vi "run.vi"(8 "error in (no error)":errorcluster, 11 "Protocol_Logging in":refnum<class "Protocol_Logging.lvclass">) -> (0 "error out":errorcluster, 3 "Protocol_Logging out":refnum<class "Protocol_Logging.lvclass">)   [LabVIEW 2011, in "Protocol_Logging.lvclass"]
uses:
  Protocol_Logging.lvclass
  protocol_Generic/Protocol_Generic.lvclass
panel:
  out "Waveform Graph":dbl[][](graph)
  out "path":path
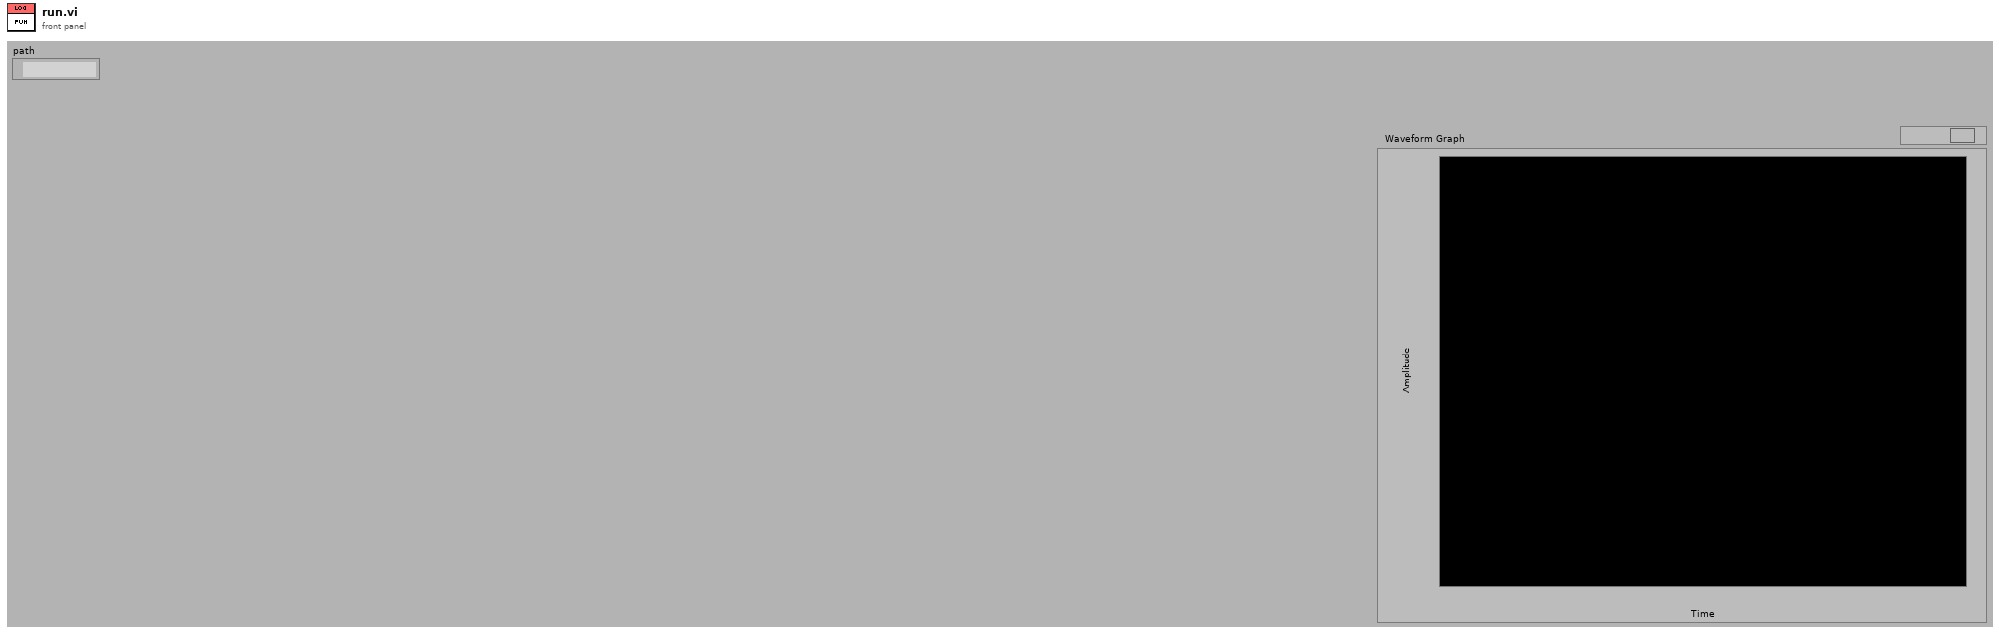
[diagram p1: front panel]
types:
  T1 = cluster{"channel0ConversionFactor":dbl, "channel1ConversionFactor":dbl, "channel2ConversionFactor":dbl}
  T2 = cluster{"Axis Information":cluster{"Device ID":i32, "Device Name":string, "Device Type":i32}[], "Axis Selector":i32[], "Control Modes out":u16[], "error out":errorcluster, "Channel Data":cluster{"Name":string, "Type":i32, "SI Full Scale":dbl, "Full Scale":dbl, "Units String":string, "Display Format":string, "Gauge Length":dbl}[][]}
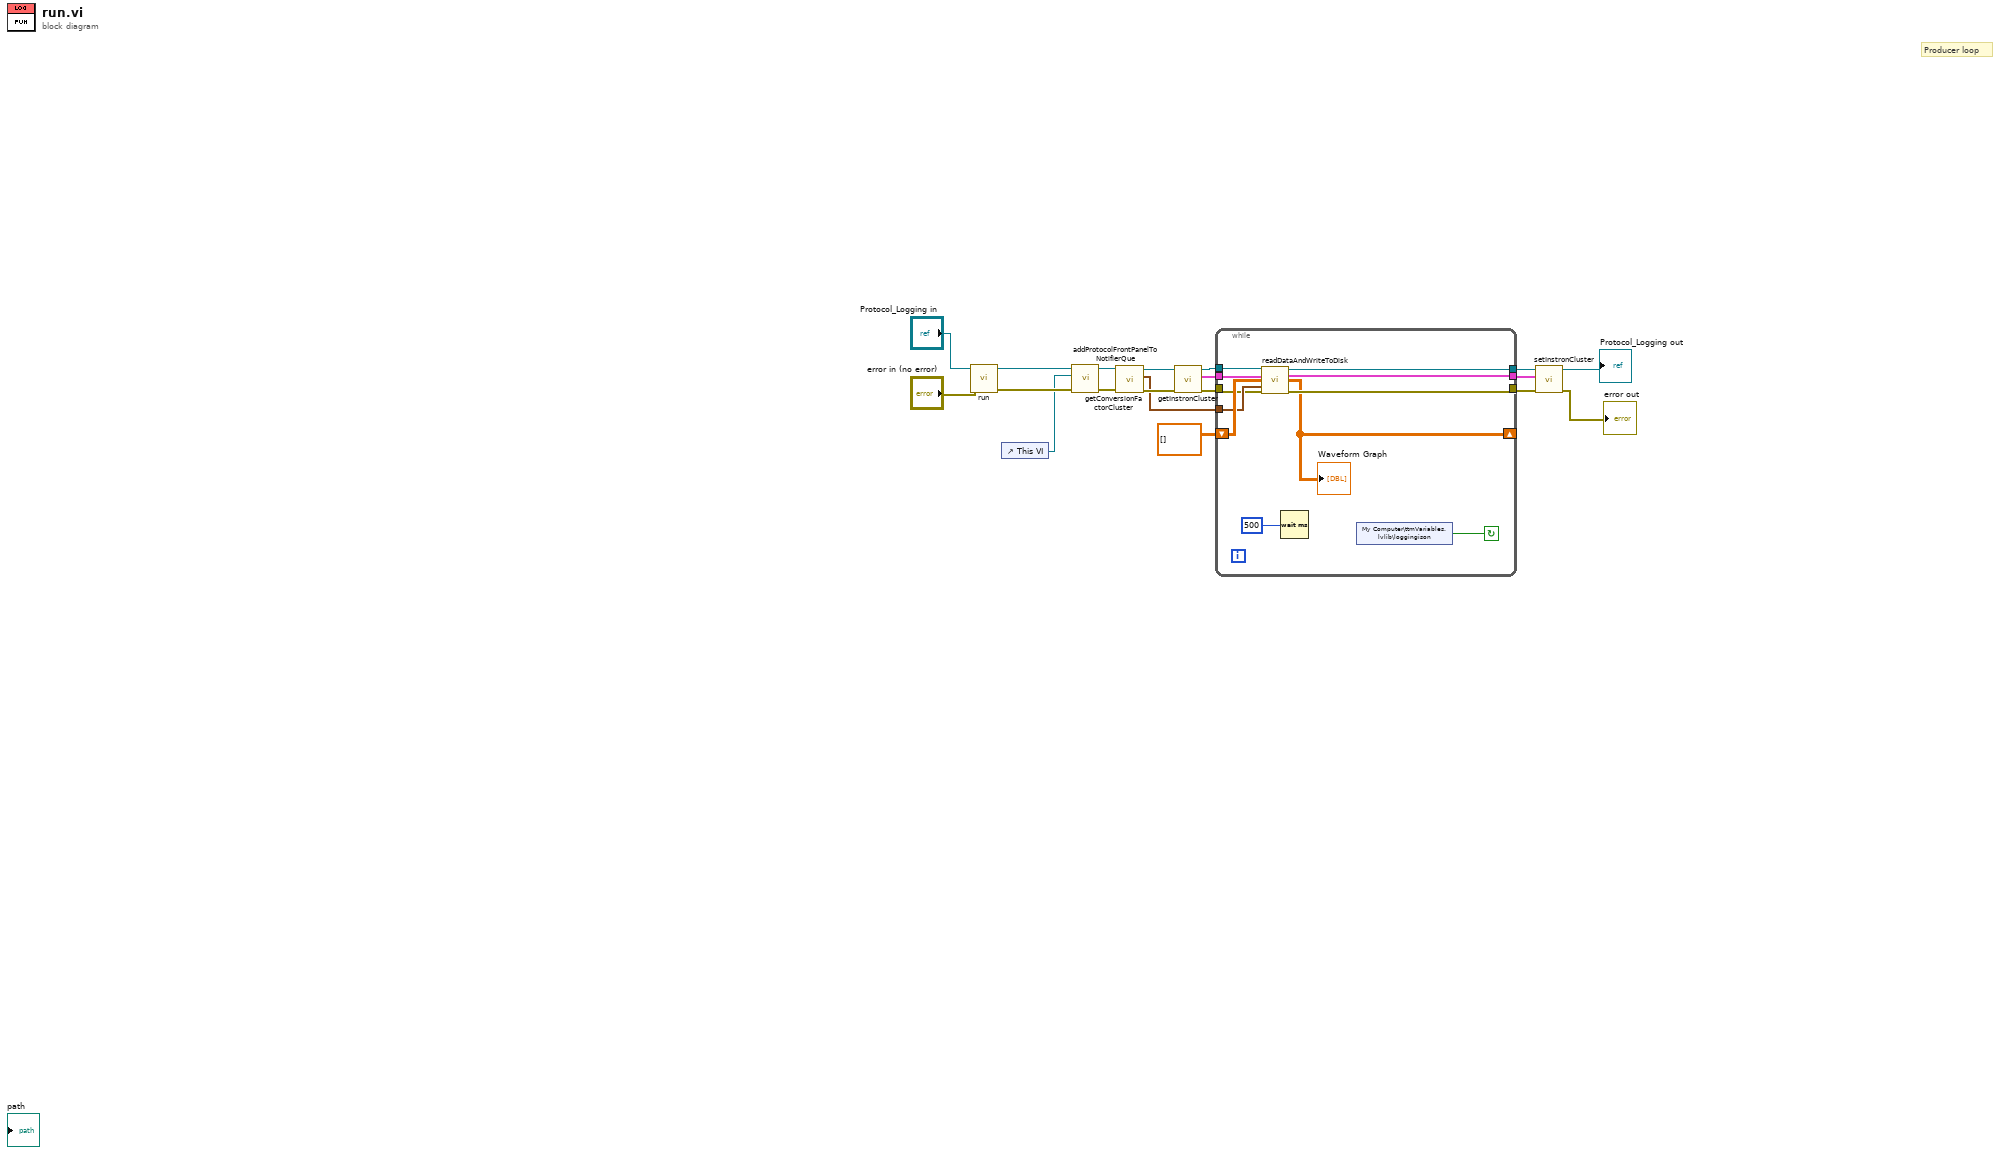
[diagram p0: block diagram]
diagram:
  # "Producer loop"
  n1 = call-parent "run.vi"("error in (no error)"="error in (no error)", "Protocol_Generic in"="Protocol_Logging in") -> ("error out"=w10:errorcluster, "Protocol_Generic out"=w11:refnum<class "Protocol_Logging.lvclass">)  [unwired: 8 in]
  n2 = control-ref of="This VI"() -> (w7:refnum<vi>)
  n3 = call-dynamic "addProtocolFrontPanelToNotifierQue.vi"("error in (no error)"=w10, "frontPanelReference"=w7, "Protocol_Generic in"=w11) -> ("error out"=w8:errorcluster, "Protocol_Generic out"=w9:refnum<class "Protocol_Logging.lvclass">)  [unwired: 7 in]
  n4 = call-dynamic "getConversionFactorCluster.vi"("error in (no error)"=w8, "Protocol_Logging in"=w9) -> ("error out"=w14:errorcluster, "conversionFactorCluster"=w2:T1, "Protocol_Logging out"=w13:refnum<class "Protocol_Logging.lvclass">)  [unwired: 6 in]
  n5 = call-dynamic "getInstronCluster.vi"("error in (no error)"=w14, "Protocol_Generic in"=w13) -> ("error out"=w1:errorcluster, "InstronCluster"=w6:T2, "Protocol_Generic out"=w5:refnum<class "Protocol_Logging.lvclass">)  [unwired: 7 in]
  n6 = while {
    tunnel: [w22] -> w17
    shift-right: [w20] -> _
    shift-left: dbl[][] [] -> [w26]
    tunnel: w6 -> [w27]
    tunnel: w5 -> [w28]
    tunnel: [w21] -> w3
    tunnel: [w23] -> w4
    tunnel: w2 -> [w25]
    tunnel: w1 -> [w24]
    stop <- w29 continue-if-true
    n7 = call-dynamic "readDataAndWriteToDisk.vi"("Protocol_Logging in"=w28, "Instron cluster in"=w27, "PreviousData"=w26, "Conversion factors"=w25, "error in (no error)"=w24) -> ("Protocol_Logging out"=w23:refnum<class "Protocol_Logging.lvclass">, "instron cluster out"=w21:T2, "CombinedDataOut"=w20:dbl[][], "error out"=w22:errorcluster)  [unwired: 7 in]
    "Waveform Graph" <- w20
    n8 = Wait (ms)(milliseconds to wait=u32 500) -> ()  [unwired: 1 out]
    n9 = shared-variable "My Computer\\ttmVariables.lvlib\\loggingison"() -> (w29:bool)  [unwired: 1 in, 1 out]
  }
  n10 = call-dynamic "setInstronCluster.vi"("error in (no error)"=w17, "InstronCluster"=w3, "Protocol_Generic in"=w4) -> ("error out"=→"error out":errorcluster, "Protocol_Generic out"=→"Protocol_Logging out":refnum<class "Protocol_Logging.lvclass">)  [unwired: 7 in]
